vi "Test Constant Elements Slices.vi"() -> ()   [LabVIEW 2021, in "Arrays.lvlib"]
uses:
  Linear Ramp End Options.ctl
  16794205-078f-4e8e-b574-4eb79d5c6cf5.vi
  Arrays.lvlib
panel:
  out "# Elements":i32=100
  out "Bin Widths":dbl[](array[numeric])=[0.09999999999999998, 0.10000000000000009, 0.10000000000000006, 0.10000000000000009, 0.10000000000000003, 0.10000000000000009, 0.09000000000000008]
  out "Bin Bounds":dbl[](array[numeric])=[0.03, 0.12999999999999998, 0.23000000000000007, 0.3300000000000001, 0.4300000000000002, 0.5300000000000002, 0.6300000000000003]
  in  "Array Stop (NaN: last)":dbl=0.78
  in  "Array Start (NaN: first)":dbl=0.03
  in  "# Elements":i32=10
  in  "Options":T1
  in  "# Steps (1)":i32=100
  in  "End (1)":dbl=1.0
  in  "Start (0)":dbl
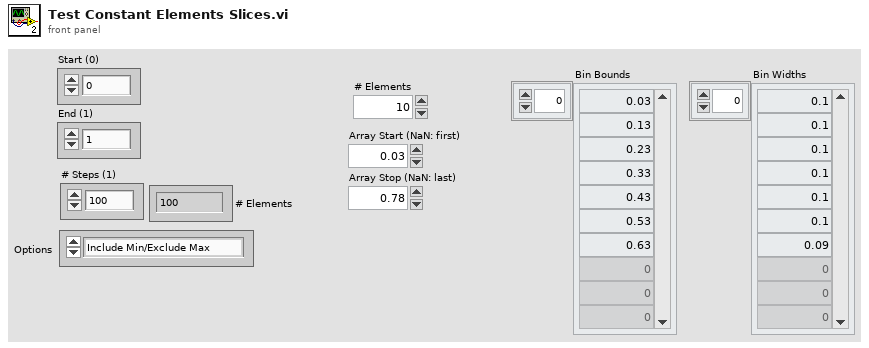
[diagram p1: front panel]
types:
  T1 = typedef "Arrays.lvlib/Linear Ramp End Options.ctl" = enum16{"Include Min/Exclude Max", "Exclude Min/Include Max", "Include Both Ends", "Exclude Both Ends"}
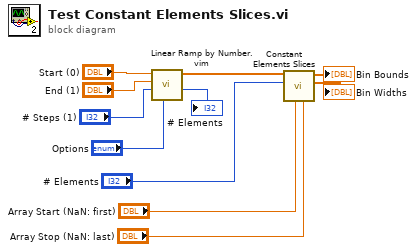
[diagram p0: block diagram]
diagram:
  n1 = call "Linear Ramp by Number.vim"("Options"="Options", "# Steps (1)"="# Steps (1)", "End (1)"="End (1)", "Start (0)"="Start (0)") -> ("# Elements"=→"# Elements":i32, "Ramp"=w7:dbl[])  [unwired: 5 in, 1 out]
  n2 = call "Constant Elements Slices.vi"("Array Stop (NaN: last)"="Array Stop (NaN: last)", "Array Start (NaN: first)"="Array Start (NaN: first)", "# Elements"="# Elements", "Sorted Array in"=w7) -> ("Bin Widths"=→"Bin Widths":dbl[], "Bin Bounds"=→"Bin Bounds":dbl[])  [unwired: 4 in, 2 out]
